vi "Get Tx Duration.vi"(8 "error in (no error)":errorcluster, 11 "Framework Performance in":refnum<class "Framework Performance.lvclass">) -> (0 "error out":errorcluster, 2 "tx duration":u32 format="%d us", 3 "Framework Performance out":refnum<class "Framework Performance.lvclass">)   [LabVIEW 2017, in "DSF Core.lvlib" / "Framework Performance.lvclass"]
uses:
  Framework Performance.lvclass
  Framework Performance.lvclass/Framework Performance.ctl
  <vilib>/NI/Memory Manager/Classes/Pointer/Pointer.lvclass/Pointer.ctl
  <vilib>/NI/Memory Manager/Classes/Pointer/Public/Read/Read (0D U32).vi
  <vilib>/NI/Memory Manager/Classes/Pointer/Public/Read (No Check)/Read (No Check 0D U32).vi
  <vilib>/NI/Memory Manager/Classes/Pointer/Protected/Parameter Checking/Check Null Pointer.vi
  <vilib>/NI/Memory Manager/Classes/Pointer/Protected/Parameter Checking/Check Subset.vi
  <vilib>/NI/Memory Manager/Classes/Pointer/API/Accessors/Get Address.vi
  <vilib>/NI/Memory Manager/Classes/Pointer/Protected/Errors.vi
  <vilib>/NI/Memory Manager/Classes/Pointer/Protected/Error VIs/Null Pointer.vi
  <vilib>/NI/Memory Manager/Classes/Pointer/Protected/Error VIs/Out of Bounds.vi
  <vilib>/NI/Memory Manager/Classes/Pointer/API/Accessors/Get Size.vi
  <vilib>/NI/Memory Manager/Classes/Pointer/Protected/Error Building/Create Error.vi
  <vilib>/NI/Memory Manager/VIs/Write String into Source.vi
  <vilib>/NI/Memory Manager/Classes/Pointer/Protected/Error Building/Write Pointer Size.vi
  <vilib>/NI/Memory Manager/VIs/Write Number into Source.vi
  <vilib>/NI/Memory Manager/VIs/VIs for Poly/Write U64 into Source.vi
  <vilib>/NI/Memory Manager/Constants/Constants.vi
  <vilib>/NI/Memory Manager/Constants/Library Name.vi
  <vilib>/NI/Memory Manager/Classes/Pointer/Protected/Error Building/Get Error Info.vi
  <vilib>/NI/Memory Manager/VIs/Create Error Cluster.vi
  <vilib>/NI/Memory Manager/VIs/VIs for Poly/Create Error Cluster (256B).vi
  <vilib>/NI/Memory Manager/VIs/Set Error Status.vi
  <vilib>/NI/Memory Manager/VIs/Set Error Code.vi
  <vilib>/NI/Memory Manager/VIs/Set Error Source.vi
  <vilib>/NI/Memory Manager/Classes/Pointer/Pointer.lvclass
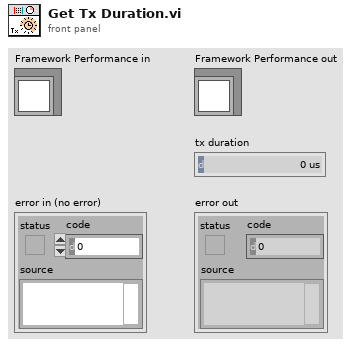
[diagram p1: front panel]
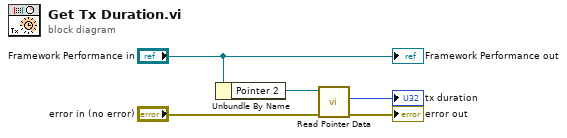
[diagram p0: block diagram]
diagram:
  n1 = Unbundle By Name("Framework Performance in") -> ("Pointer 2"=w5:refnum<class "Pointer.lvclass">)
  n2 = call-poly <vilib>:"Read Pointer Data.vi"("error in (no error)"="error in (no error)", "Pointer in"=w5) -> ("error out"=→"error out":errorcluster, "value out"=→"tx duration":u32)  [unwired: 6 in, 2 out]
  "Framework Performance out" <- "Framework Performance in"
